vi "destroy.vi"(8 "error in (no error)":errorcluster, 11 "ExampleTask_StopNotifier in":refnum<class "ExampleTask_StopNotifier.lvclass">) -> (0 "error out":errorcluster, 3 "loopCounter":i32)   [LabVIEW 2023, in "ExampleTask_StopNotifier.lvclass"]
doc: "Destructor.\nIt also returns the value of loopCounter."
uses:
  ExampleTask_StopNotifier.lvclass
  ExampleTask_StopNotifier.lvclass/ExampleTask_StopNotifier.ctl
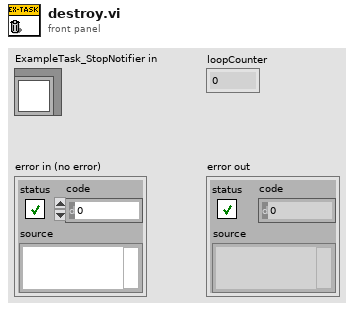
[diagram p1: front panel]
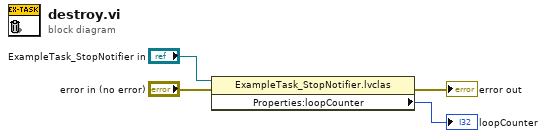
[diagram p0: block diagram]
diagram:
  n1 = property class="ExampleTask_StopNotifier.lvclas"(reference="ExampleTask_StopNotifier in", error in="error in (no error)") -> (error out=→"error out":errorcluster, "Properties:loopCounter"=→"loopCounter":i32)  [unwired: 1 out]
